vi "Read Recording Error File Write Cells.vi"(5 "Reason Column Letter":string="D", 7 "Depth Column Letter":string="C", 8 "error in (no error)":errorcluster, 9 "Row Offset In":i32, 10 "Sonde Data file":path, 11 "NI_report in":refnum<class "NI_report.lvclass">) -> (0 "error out":errorcluster, 1 "all rows":string[][](array[string]), 2 "Row Offset Out":i32, 3 "NI_report out":refnum<class "NI_report.lvclass">)   [LabVIEW 2016]
uses:
  <vilib>/Utility/NIReport.llb/NI_report.lvclass
  <vilib>/Utility/file.llb/Read Delimited Spreadsheet (string).vi
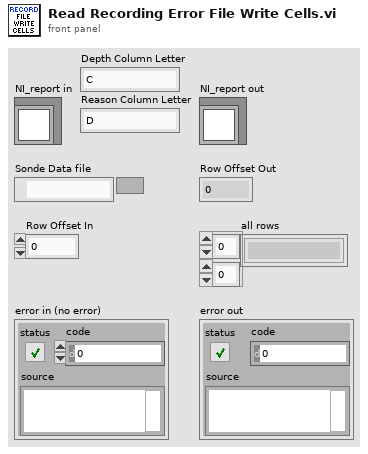
[diagram p1: front panel]
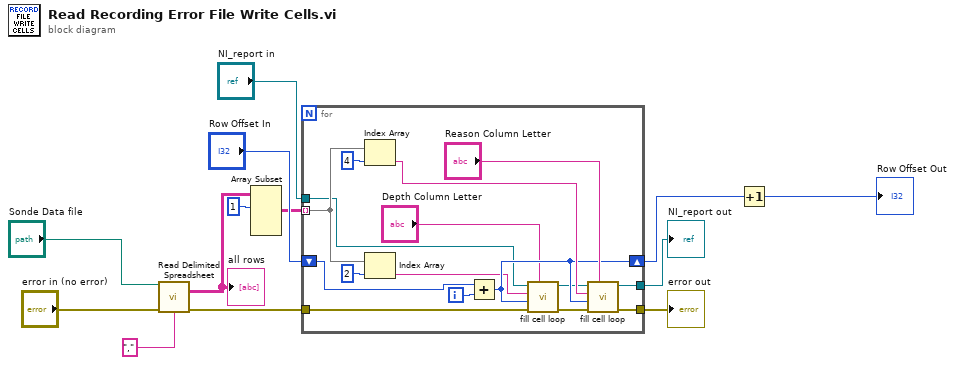
[diagram p0: block diagram]
diagram:
  n1 = call-poly <vilib>:"Read Delimited Spreadsheet.vi"("file path (dialog if empty)"="Sonde Data file", "error in (no error)"="error in (no error)", "delimiter (\\t)"="," ("delimiter (\\t)")) -> ("all rows"=w4:string[][], "error out"=w13:errorcluster)  [unwired: 7 in, 4 out]
  "all rows" <- w4
  n2 = Array Subset(array=w4, index (row)=1 ("index")) -> (w6:string[][])  [unwired: 3 in]
  n3 = for {
    tunnel: w6 -> [w21] mode=indexing
    shift-right: [w18] -> w9
    shift-left: "Row Offset In" -> [w29]
    tunnel: "NI_report in" -> [w16]
    tunnel: w13 -> [w20]
    tunnel: [w26] -> w11
    tunnel: [w25] -> w10
    i -> [w28]
    n4 = Index Array(array=w21, index=4) -> (element=w22:string)
    n5 = Index Array(array=w21, index=2) -> (element=w17:string)
    n6 = Add(x=w29, y=w28) -> (x+y=w18:i32)
    n7 = call "fill cell loop.vi"("Column Letter"="Depth Column Letter", "error in (no error)"=w20, "Row"=w18, "String"=w17, "NI_report in"=w16) -> ("error out"=w19:errorcluster, "NI_report out"=w15:refnum<class "NI_report.lvclass">)  [unwired: 5 in]
    n8 = call "fill cell loop.vi"("Column Letter"="Reason Column Letter", "error in (no error)"=w19, "Row"=w18, "String"=w22, "NI_report in"=w15) -> ("error out"=w26:errorcluster, "NI_report out"=w25:refnum<class "NI_report.lvclass">)  [unwired: 5 in]
  }
  "error out" <- w11
  "NI_report out" <- w10
  n9 = Increment(x=w9) -> (x+1=→"Row Offset Out":i32)
